vi "MainRT.vi"() -> ()   [LabVIEW 2017]
doc: "The myRIO Project template acquires acceleration data from the onboard accelerometer and displays the changes of acceleration values in a waveform chart."
uses:
  TypeDefs/CommandsRT.ctl
  Projekt-RubikLibrary/OrientationState.ctl
  Projekt-RubikLibrary/RubikMoves.ctl
  <extravilib>/ChannelInstances/Stream-t'DataStreamCluster.ctl'/Read With Abort.vi
  <extravilib>/ChannelInstances/Stream-t'DataStreamCluster.ctl'/Write With Abort.vi
  <vilib>/myRIO/Common/Instrument Driver Framework/myRIO v1.0/UART/vis/myRIO v1.0 Close UART.vi
  <extravilib>/ChannelInstances/Stream-t'DataStreamCluster.ctl'/EndpointRead.vi
  <extravilib>/ChannelInstances/Stream-t'DataStreamCluster.ctl'/Endpoint.vi
  <extravilib>/ChannelInstances/Stream-t'DataStreamCluster.ctl'/Instantiate.vi
  <extravilib>/ChannelInstances/Stream-t'DataStreamCluster.ctl'/)Channel.vi
  <resource>/ChannelSupport/_ChannelSupport/WaitIfNeeded.vi
  <vilib>/myRIO/Common/Instrument Driver Framework/Utilities/vis/FPGA Ref Manager.vi
  <vilib>/myRIO/Common/Instrument Driver Framework/myRIO v1.0/myRIO v1.0 Reset FPGA.vi
  <vilib>/myRIO/Common/Instrument Driver Framework/myRIO v1.0/IRQ/vis/myRIO v1.0 IRQ Info FGV.vi
  <vilib>/myRIO/Common/Instrument Driver Framework/myRIO v1.0/IRQ/vis/myRIO v1.0 Timer IRQ Info FGV.vi
  <vilib>/myRIO/Common/Instrument Driver Framework/myRIO v1.0/IRQ/vis/myRIO v1.0 ISR Agent.vi
  <vilib>/myRIO/Instrument Drivers/Utilities/Utilities.lvlib
  <extravilib>/ChannelInstances/Stream-t'DataStreamCluster.ctl'.lvlib
  Projekt-RubikLibrary/RubikLibraryRT.lvlib
  Projekt-RubikLibrary/RubikLibrary.lvlib
panel:
  out "Final Orientation":T1
  out "Command":T2
  out "error out":errorcluster
  # "Overview  MainRT\n\nRotate the Cube!\n\nMainRT on myRIO receives commands from PC via Network Streams.\nMainPC sends the commands."
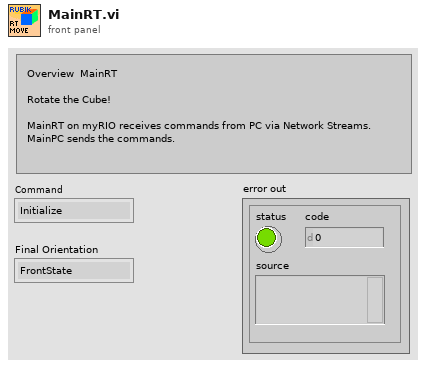
[diagram p1: front panel]
types:
  T1 = typedef "RubikLibrary.lvlib/OrientationState.ctl" = enum16{"FrontState", "UpState", "BackState", "DownState"}
  T2 = typedef "CommandsRT.ctl" = enum16{"Initialize", "Rotate", "Exit"}
  T3 = typedef "DataStreamCluster.ctl" = cluster{"Commands":T2, "Variant":variant}
  T4 = typedef "Stream-t'DataStreamCluster.ctl'.lvlib/)Channel.ctl" = refnum<queue>
  T5 = typedef "RubikLibrary.lvlib/RubikMoves.ctl" = enum16{"U", "U'", "F", "F'", "D", "D'", "B", "B'", "L", "L'", "R", "R'"}
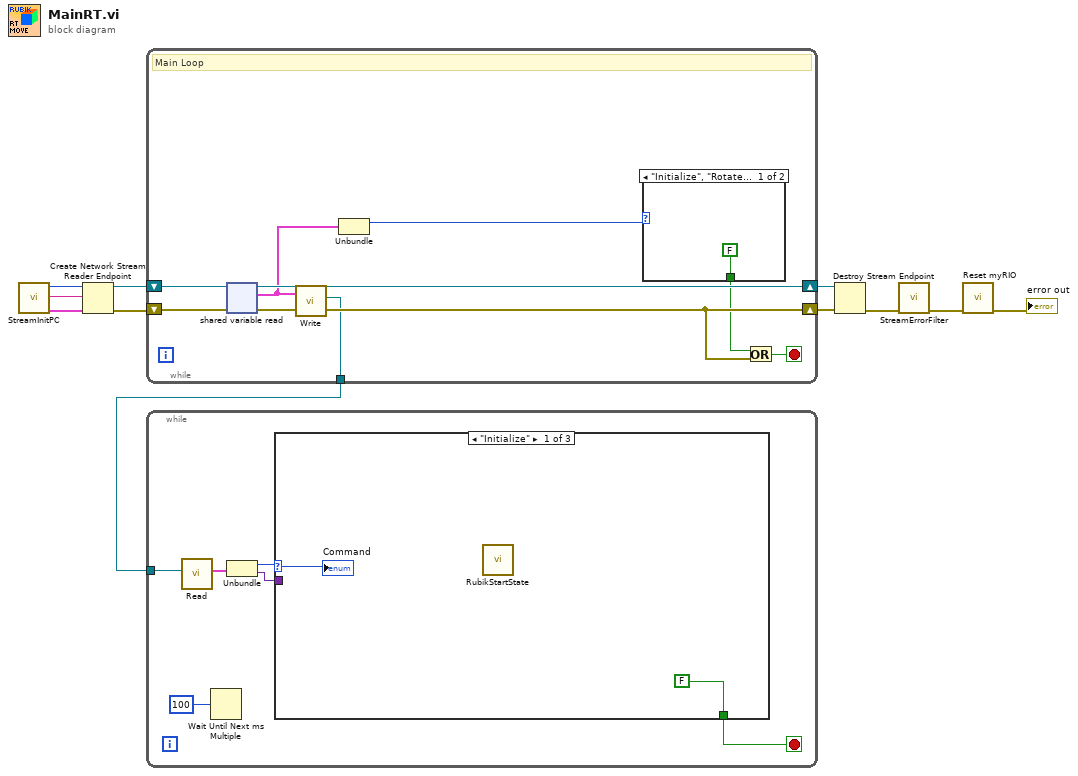
[diagram p0: block diagram]
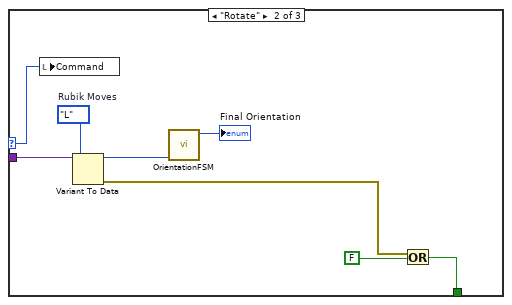
[diagram p2: hidden frame]
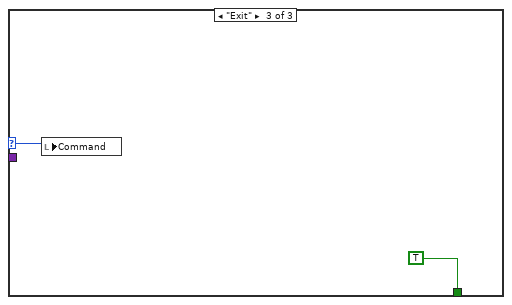
[diagram p3: hidden frame]
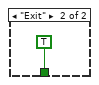
[diagram p4: hidden frame]
diagram:
  n1 = call "StreamInitPC.vi"() -> ("data cluster"=w4:T3, "reader name"=w11:string, "writer buffer size"=w10:i32)  [unwired: 4 in, 1 out]
  n2 = Create Network Stream Reader Endpoint(7:w10, 9:w4, 11:w11) -> (0:w9:errorcluster, 3:w8:refnum<k21>)  [unwired: 4 in]
  n3 = while {
    shift-right: [w18] -> w5
    shift-left: w9 -> [w18]
    shift-right: [w16] -> w6
    shift-left: w8 -> [w17]
    tunnel: [w13] -> w1
    stop <- w19 stop-if-true
    # "Main Loop"
    n4 = shared-variable-read(w17) -> (w16:refnum<k21>, w14:T3)  [unwired: 2 in, 2 out]
    n5 = call <extravilib>:"Write.vi"("element"=w14) -> ("channel"=w13:T4)  [unwired: 8 in, 2 out]
    n6 = Unbundle(w14) -> ("Commands"=w12:T2)  [unwired: 1 out]
    n7 = case shown="\"Initialize\", \"Rotate\"" w12 {
      tunnel: [FALSE TRUE] -> w15
      frame "Initialize", "Rotate" {
      }
      frame "Exit" {
      }
    }
    n8 = Or(x=w15, y=w18) -> (x .or. y?=w19:bool)
  }
  n9 = while {
    tunnel: w1 -> [w25]
    stop <- w27 stop-if-true
    n10 = call <extravilib>:"Read.vi"("channel"=w25) -> ("element"=w24:T3)  [unwired: 6 in, 4 out]
    n11 = Wait Until Next ms Multiple(millisecond multiple=u32 100) -> ()  [unwired: 1 out]
    n12 = Unbundle(w24) -> ("Commands"=w23:T2, "Variant"=w22:variant)
    n13 = case shown="\"Initialize\"" w23 {
      selector: w23 -> [w29 w37 w39]
      tunnel: [FALSE w30 TRUE] -> w27
      tunnel: w22 -> [_ w33 _]
      frame "Initialize" {
        n14 = call "RubikStartState.vi"() -> ()  [unwired: 11 in, 1 out]
        "Command" <- w29
      }
      frame "Rotate" {
        w36 = RubikMoves."L"  # Rubik Moves
        n15 = local write "Command"(w37) -> ()
        n16 = Variant To Data(type=w36, Variant=w33) -> (data=w35:T5, error out=w32:errorcluster)  [unwired: 1 in]
        n17 = call "OrientationFSM.vi"("Rubik's Moves"=w35) -> ("Final Orientation"=→"Final Orientation":T1)  [unwired: 10 in]
        n18 = Or(x=w32, y=FALSE) -> (x .or. y?=w30:bool)
      }
      frame "Exit" {
        n19 = local write "Command"(w39) -> ()
      }
    }
  }
  n20 = Destroy Stream Endpoint(8:w5, 11:w6) -> (0:w7:errorcluster)
  n21 = call "StreamErrorFilter.vi"("error in (no error)"=w7) -> ("error out"=w2:errorcluster)  [unwired: 10 in]
  n22 = call <vilib>:"Reset myRIO.vi"("error in (no error)"=w2) -> ("error out"=→"error out":errorcluster)  [unwired: 10 in]
